vi "MKS.vi"(9 "IP Array":string[](array[string]), 10 "Connect":bool) -> (2 "Emissions":dbl[](array[numeric]))   [LabVIEW 2014]
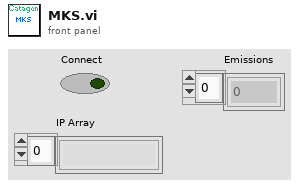
[diagram p1: front panel]
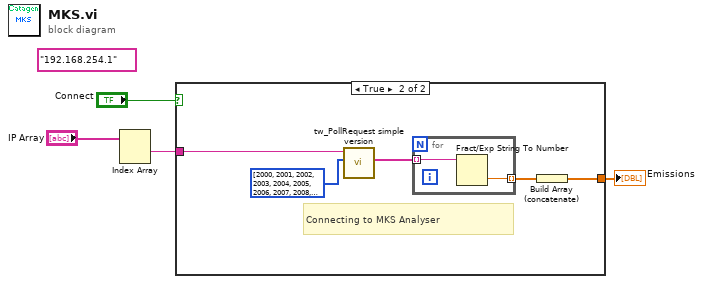
[diagram p0: block diagram]
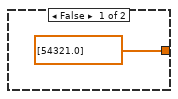
[diagram p2: hidden frame]
diagram:
  (unwired) "192.168.254.1" ("IP_ADD [127.0.0.1]")
  n1 = Index Array(array="IP Array") -> (element #1=w1:string)  [unwired: 2 in, 1 out]
  n2 = case shown="True" "Connect" {
    tunnel: w1 -> [_ w7]
    tunnel: [dbl[] [54321.0] w6] -> w4
    frame False {
    }
    frame True {
      # "Connecting to MKS Analyser"
      n3 = call <userlib>:"tw_PollRequest simple version.vi"("EVID list"=i32[] [2000, 2001, 2002, 2003, 2004, 2005, 2006, 2007, 2008, 2009, 2010, 2011, 2012, 2014, 2015], "IP_ADD [127.0.0.1]"=w7) -> ("values out"=w8:string[])  [unwired: 7 in, 2 out]
      n4 = for {
        tunnel: [w12] -> w10 mode=indexing
        tunnel: w8 -> [w11] mode=indexing
        n5 = Fract/Exp String To Number(string=w11) -> (number=w12:dbl)  [unwired: 3 in, 1 out]
      }
      n6 = Build Array (concatenate)(w10) -> (w6:dbl[])
    }
  }
  "Emissions" <- w4
